vi "get_data_block.vi"(7 "circular mode?":bool, 8 "error in (no error)":errorcluster, 11 "DAQmxWriteSignals in":refnum<class "SignalWriterDL090202DAQmx.lvclass">) -> (0 "error out":errorcluster, 2 "data block":dbl[][](array[numeric]), 3 "DAQmxWriteSignals out":refnum<class "SignalWriterDL090202DAQmx.lvclass">, 4 "actual block size (samples)":i32, 6 "current offset (samples)":i32)   [LabVIEW 2010, in "SignalWriterDL090202DAQmx.lvclass"]
uses:
  SignalWriterDL090202DAQmx.lvclass
  GenericSignalWriter/GenericSignalWriter/GenericSignalWriter.lvclass
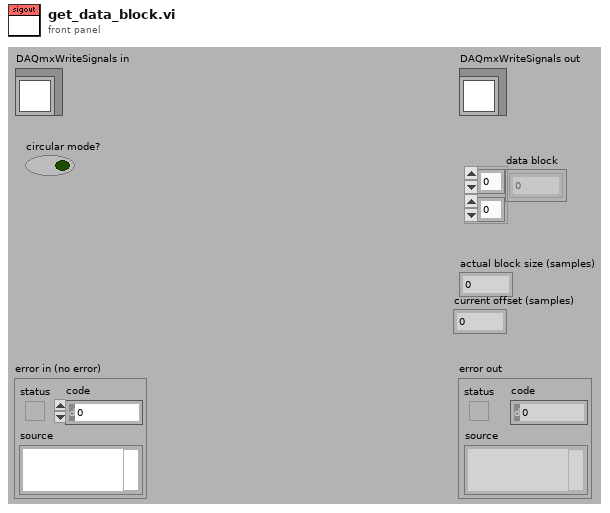
[diagram p1: front panel]
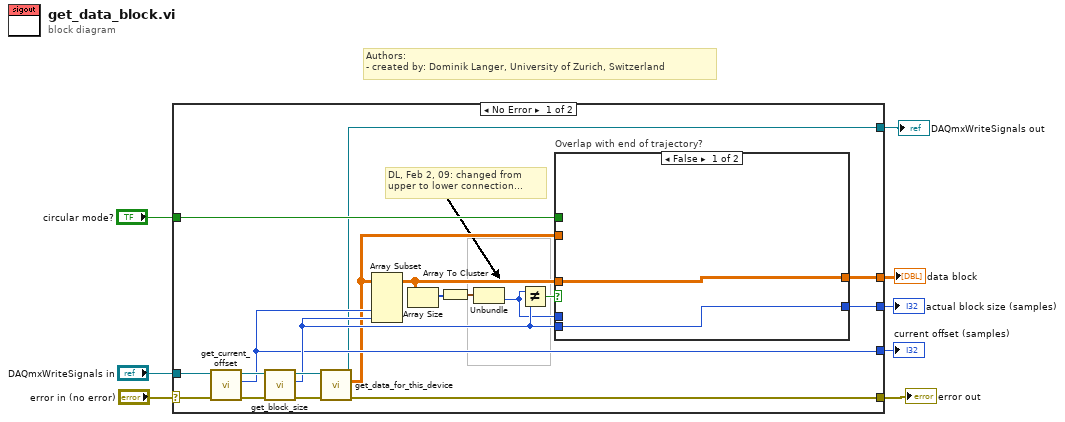
[diagram p0: block diagram]
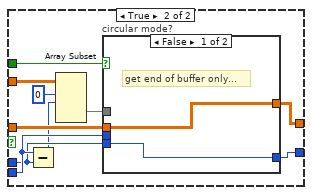
[diagram p2: hidden frame]
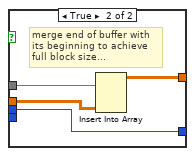
[diagram p3: hidden frame]
diagram:
  # "Authors: \n- created by: Dominik Langer, University of Zurich, Switzerland"
  n1 = case shown="No Error" "error in (no error)" {
    selector: "error in (no error)" -> [w27 w47]
    tunnel: [w21 w47] -> w7
    tunnel: [w10 w46] -> w5
    tunnel: "DAQmxWriteSignals in" -> [w26 w46]
    tunnel: "circular mode?" -> [w16 _]
    tunnel: [w15 _] -> w3
    tunnel: [w14 _] -> w2
    tunnel: [w12 _] -> w1
    frame No Error {
      # "DL, Feb 2, 09: changed from\nupper to lower connection..."
      n2 = call-dynamic "get_current_offset.vi"("error in (no error)"=w27, "GenericWriteSignals.lvclass in"=w26) -> ("error out"=w24:errorcluster, "current offset (samples)"=w12:i32, "GenericWriteSignals.lvclass out"=w25:refnum<class "SignalWriterDL090202DAQmx.lvclass">)  [unwired: 7 out]
      n3 = call "get_block_size.vi"("error in (no error)"=w24, "GenericWriteSignals.lvclass in"=w25) -> ("error out"=w22:errorcluster, "block size"=w13:i32, "GenericWriteSignals.lvclass out"=w23:refnum<class "SignalWriterDL090202DAQmx.lvclass">)  [unwired: 7 out]
      n4 = call-dynamic "get_data_for_this_device.vi"("error in (no error)"=w22, "DAQmxWriteSignals in"=w23) -> ("error out"=w21:errorcluster, "data"=w11:dbl[][], "DAQmxWriteSignals out"=w10:refnum<class "SignalWriterDL090202DAQmx.lvclass">)  [unwired: 7 out]
      n5 = Array Subset(array=w11, index (col)=w12, length (col)=w13) -> (w20:dbl[][])  [unwired: 2 in]
      n6 = Array Size(array=w20) -> (size(s)=w18:i32[])
      n7 = Array To Cluster(array=w18) -> (cluster=w17:cluster{"[0]":i32, "[1]":i32})
      n8 = Unbundle(w17) -> ("[1]"=w9:i32)  [unwired: 1 out]
      n9 = Not Equal?(x=w9, y=w13) -> (x != y?=w19:bool)
      n10 = case "Overlap with end of trajectory?" shown="False" w19 {
        tunnel: w11 -> [_ w39]
        tunnel: w13 -> [w28 w32]
        tunnel: w20 -> [w29 w37]
        tunnel: [w29 w35] -> w15
        tunnel: w9 -> [_ w31]
        tunnel: w16 -> [_ w34]
        tunnel: [w28 w33] -> w14
        frame False {
        }
        frame True {
          n11 = Subtract(x=w32, y=w31) -> (x-y=w30:i32)
          n12 = Array Subset(array=w39, index (row)=0 ("index"), length (row)=w30) -> (w36:dbl[][])  [unwired: 2 in]
          n13 = case "circular mode?" shown="False" w34 {
            tunnel: w37 -> [w41 w42]
            tunnel: w36 -> [_ w44]
            tunnel: [w41 w43] -> w35
            tunnel: [w40 w45] -> w33
            tunnel: w32 -> [_ w45]
            tunnel: w31 -> [w40 _]
            frame False {
              # "get end of buffer only..."
            }
            frame True {
              # "merge end of buffer with its beginning to achieve full block size..."
              n14 = Insert Into Array(array=w44, new element=w42) -> (w43:dbl[][])  [unwired: 2 in]
            }
          }
        }
      }
    }
    frame Error {
    }
  }
  "error out" <- w7
  "DAQmxWriteSignals out" <- w5
  "data block" <- w3
  "actual block size (samples)" <- w2
  "current offset (samples)" <- w1
